vi "Test Add Sheet with empty name.vi"(11 "Test Case In":refnum<class "Test Open Xml.lvclass">) -> (0 "error out":errorcluster, 3 "Test Case Out":refnum<class "Test Open Xml.lvclass">)   [LabVIEW 2020, in "Test Open Xml.lvclass"]
uses:
  Test Open Xml.lvclass
  C:/Program Files/National Instruments/LabVIEW 2025/vi.lib/Astemes/LUnit/Test Case.lvclass
  <vilib>/Astemes/LUnit/Test Case.lvclass/Test Case.ctl
  3fd9ecb3-cb99-4db2-8a80-5e80f6af10ae.vi
  <vilib>/Astemes/LUnit/Core/LUnit Test Case/Private/Append Pass Result.vi
  <vilib>/Astemes/LUnit/Core/LUnit Test Case/Private/Append Fail Result.vi
  3fd9ecb3-cb99-4db2-8a80-5e80f6af10ae.vi/9c5d11cd-9439-4240-a1ee-d9baace9c924.vi
  <vilib>/Astemes/LUnit/Core/LUnit Test Case/Private/Run In UI.vi
  <vilib>/Utility/error.llb/Clear Errors.vi
  Source/Open Xml.lvlib
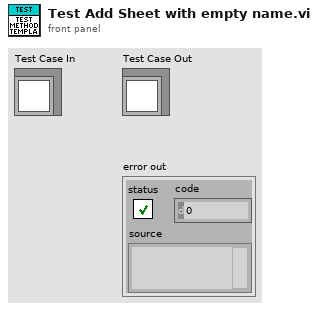
[diagram p1: front panel]
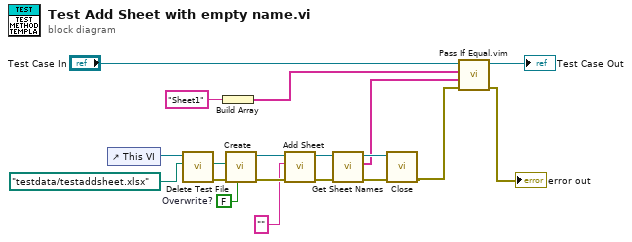
[diagram p0: block diagram]
diagram:
  w3 = FALSE  # Overwrite?
  n1 = control-ref of="This VI"() -> (w6:refnum<vi>)
  n2 = call "Delete Test File.vi"("name or relative path"=path "testdata/testaddsheet.xlsx", "VI in"=w6) -> ("error out"=w5:errorcluster, "deleted path"=w4:path)  [unwired: 8 in]
  n3 = Build Array("Sheet1" ("SheetName")) -> (w1:string[])
  n4 = call "Create.vi"("Overwrite?"=w3, "error in"=w5, "Path"=w4) -> ("error out"=w16:errorcluster, "SpreadsheetDoc"=w14:refnum<k24>)  [unwired: 7 in]
  n5 = call "Add Sheet.vi"("error in"=w16, "Sheet Name in"="" ("SheetName"), "SpreadsheetDoc in"=w14) -> ("error out"=w15:errorcluster, "SpreadsheetDoc out"=w11:refnum<k24>)  [unwired: 6 in, 1 out]
  n6 = call "Get Sheet Names.vi"("error in"=w15, "SpreadsheetDoc in"=w11) -> ("error out"=w12:errorcluster, "Sheet Names"=w9:string[], "SpreadsheetDoc out"=w10:refnum<k24>)  [unwired: 7 in]
  n7 = call "Close.vi"("error in"=w12, "SpreadsheetDoc"=w10) -> ("error out"=w13:errorcluster)  [unwired: 9 in]
  n8 = call "Pass If Equal.vim"("error in (no error)"=w13, "Actual"=w9, "Expected"=w1, "LUnit Test Case In"="Test Case In") -> ("error out"=→"error out":errorcluster, "LUnit Test Case Out"=→"Test Case Out":refnum<class "Test Open Xml.lvclass">)  [unwired: 6 in]
